vi "OP300ZP_ADJ.vi"(8 "errin":errorcluster caption="entrée d'erreur (pas d'erreur)", 10 "BT3562A":string(combo) caption="Nom de ressource VISA") -> (0 "errout":errorcluster caption="sortie d'erreur", 2 "ADJ?":bool)   [LabVIEW 2020]
uses:
  <vilib>/Instr/_visa.llb/VISA Configure Serial Port (Instr).vi
panel:
  out "OUT 2":string
  out "OUT":string
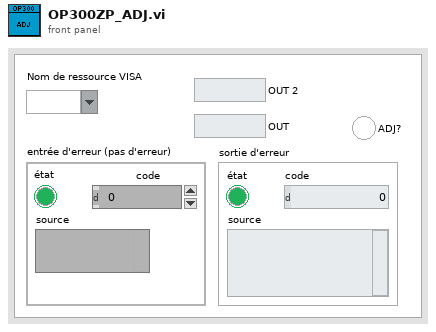
[diagram p1: front panel]
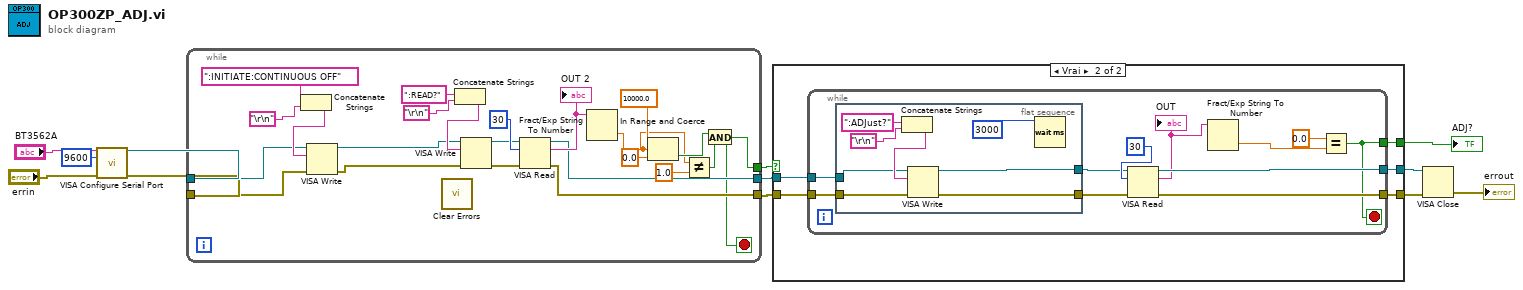
[diagram p0: block diagram]
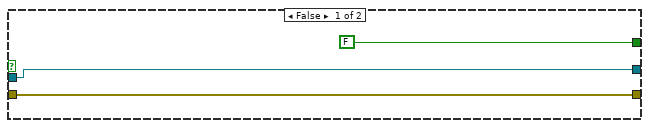
[diagram p2: hidden frame]
diagram:
  n1 = call-poly "VISA Configure Serial Port"("VISA resource name"="BT3562A", "baud rate (9600)"=u32 9600, "error in (no error)"="errin") -> ("VISA resource name out"=w4:refnum<visa-resource-name>, "error out"=w3:errorcluster)  [unwired: 11 in]
  n2 = while {
    tunnel: [w13] -> w5
    tunnel: w4 -> [w22]
    tunnel: w3 -> [w23]
    tunnel: [w28] -> w2
    tunnel: [w27] -> w1
    stop <- w13 stop-if-true
    n3 = Concatenate Strings(":INITIATE:CONTINUOUS OFF" ("buffer d'écriture"), "\r\n") -> (w24:string)
    n4 = VISA Write(VISA resource name=w22, write buffer=w24, error in (no error)=w23) -> (VISA resource name out=w20:refnum<visa-resource-name>, error out=w21:errorcluster)  [unwired: 1 out]
    n5 = call <vilib>:"Clear Errors.vi"() -> ()  [unwired: 6 in, 2 out]
    n6 = Concatenate Strings(":READ?" ("buffer d'écriture"), "\r\n") -> (w31:string)
    n7 = VISA Write(VISA resource name=w20, write buffer=w31, error in (no error)=w21) -> (VISA resource name out=w34:refnum<visa-resource-name>, error out=w30:errorcluster)  [unwired: 1 out]
    n8 = VISA Read(VISA resource name=w34, byte count=u32 30 ("nombre d'octets"), error in (no error)=w30) -> (VISA resource name out=w27:refnum<visa-resource-name>, read buffer=w29:string, error out=w28:errorcluster)  [unwired: 1 out]
    "OUT 2" <- w29
    n9 = Fract/Exp String To Number(string=w29) -> (number=w15:dbl)  [unwired: 3 in, 1 out]
    n10 = In Range and Coerce(upper limit=10000.0 ("limite supérieure"), x=w15, lower limit=0.0 ("limite inférieure")) -> (In Range?=w17:bool)  [unwired: 1 out]
    n11 = Not Equal?(x=w15, y=1.0) -> (x != y?=w14:bool)
    n12 = And(x=w17, y=w14) -> (x .and. y?=w13:bool)
  }
  n13 = case shown="Vrai" w5 {
    tunnel: [FALSE w43] -> w12
    tunnel: [w37 w42] -> w11
    tunnel: [w38 w41] -> w10
    tunnel: w2 -> [w38 w40]
    tunnel: w1 -> [w37 w39]
    frame False {
    }
    frame True {
      n14 = while {
        tunnel: [w47] -> w43
        tunnel: [w51] -> w41
        tunnel: [w50] -> w42
        tunnel: w40 -> [w49]
        tunnel: w39 -> [w48]
        stop <- w47 stop-if-true
        n15 = flat-sequence {
          tunnel: w49 -> [w57]
          tunnel: w48 -> [w56]
          tunnel: [w62] -> w54
          tunnel: [w61] -> w52
          frame #0 {
            n16 = Concatenate Strings(":ADJust?" ("buffer d'écriture"), "\r\n") -> (w58:string)
            n17 = VISA Write(VISA resource name=w56, write buffer=w58, error in (no error)=w57) -> (VISA resource name out=w61:refnum<visa-resource-name>, error out=w62:errorcluster)  [unwired: 1 out]
            n18 = Wait (ms)(milliseconds to wait=u32 3000 ("attente (ms)")) -> ()  [unwired: 1 out]
          }
        }
        n19 = VISA Read(VISA resource name=w52, byte count=u32 30 ("nombre d'octets"), error in (no error)=w54) -> (VISA resource name out=w50:refnum<visa-resource-name>, read buffer=w46:string, error out=w51:errorcluster)  [unwired: 1 out]
        "OUT" <- w46
        n20 = Fract/Exp String To Number(string=w46) -> (number=w45:dbl)  [unwired: 3 in, 1 out]
        n21 = Equal?(x=0.0, y=w45) -> (x = y?=w47:bool)
      }
    }
  }
  "ADJ?" <- w12
  n22 = VISA Close(VISA resource name=w11, error in (no error)=w10) -> (error out=→"errout":errorcluster)
